vi "AB_820_850_Project_DLL_Info.vi"(7 "action":T1, 8 "error in (no error)":errorcluster, 10 "Dll_info in":T2, 11 "Object In":T3) -> (0 "error out":errorcluster, 2 "Dll info out":T2, 3 "Object Out":T3)   [LabVIEW 2020]
uses:
  <resource>/Framework/Providers/API/ItemRef.ctl
  <vilib>/AppBuilder/RW_Project/AB_RW_Project_PropBag_Action.ctl
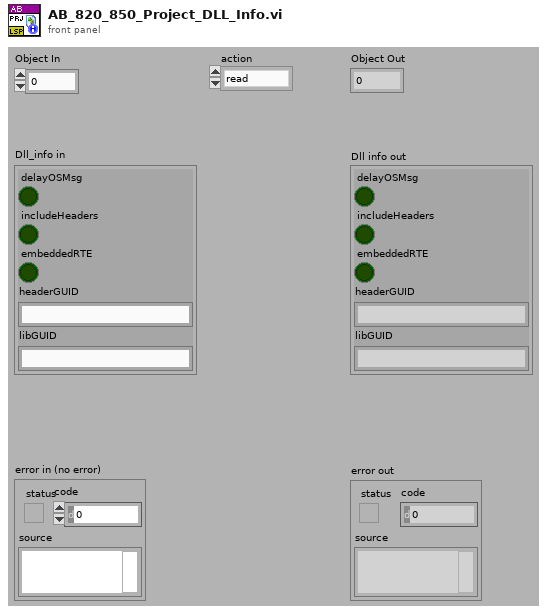
[diagram p1: front panel]
types:
  T1 = typedef "AB_RW_Project_PropBag_Action.ctl" = enum16{"read", "write", "clear", "readPrevious", "writePrevious", "clearPrevious"}
  T2 = cluster{"delayOSMsg":bool, "includeHeaders":bool, "embeddedRTE":bool, "headerGUID":string, "libGUID":string}
  T3 = typedef "ItemRef.ctl" = u64
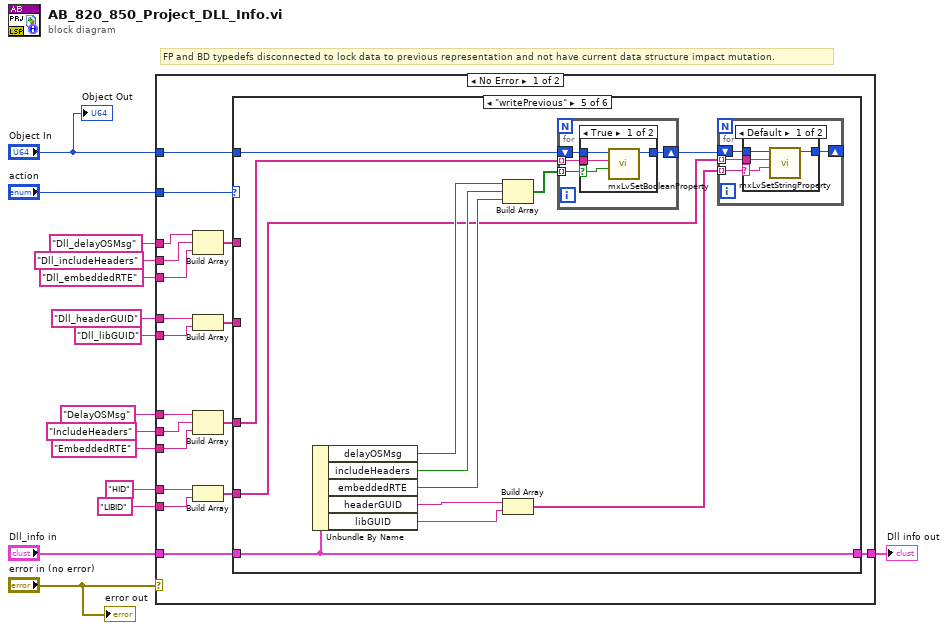
[diagram p0: block diagram]
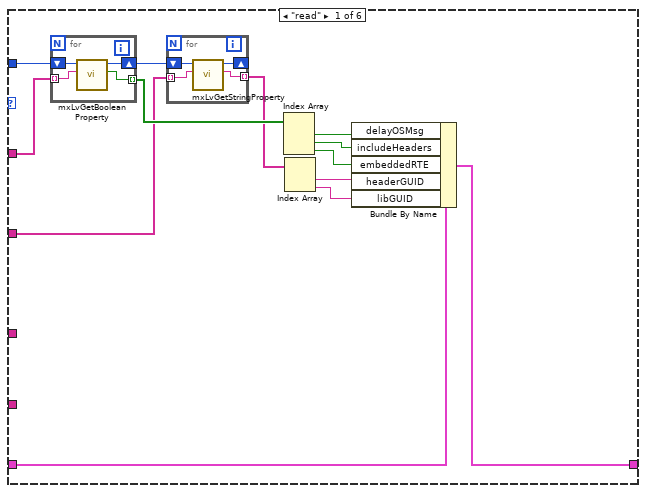
[diagram p2: hidden frame]
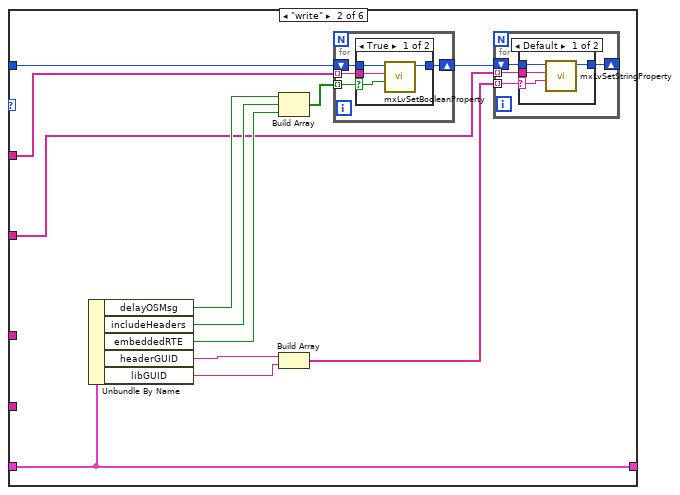
[diagram p3: hidden frame]
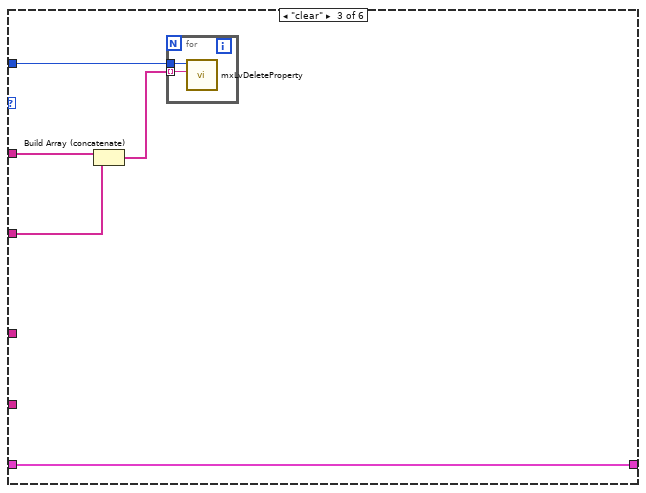
[diagram p6: hidden frame]
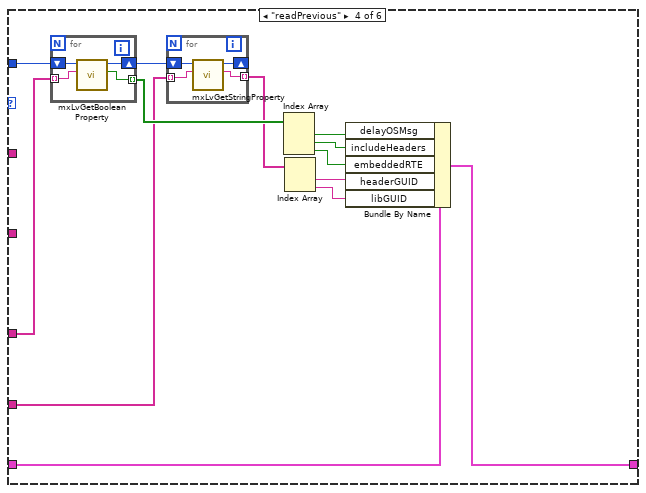
[diagram p7: hidden frame]
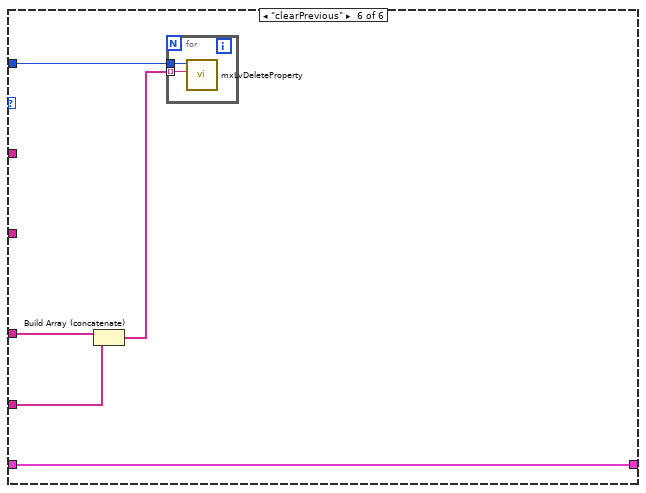
[diagram p10: hidden frame]
diagram:
  # "FP and BD typedefs disconnected to lock data to previous representation and not have current data structure impact mutation."
  n1 = case shown="No Error" "error in (no error)" {
    tunnel: "Object In" -> [w32 _]
    tunnel: [w33 _] -> w13
    tunnel: "Dll_info in" -> [w31 _]
    tunnel: "action" -> [w30 _]
    tunnel: "DelayOSMsg" -> [w29 _]
    tunnel: "IncludeHeaders" ("Tag") -> [w28 _]
    tunnel: "EmbeddedRTE" ("Tag") -> [w27 _]
    tunnel: "HID" -> [w25 _]
    tunnel: "LIBID" -> [w24 _]
    tunnel: "Dll_delayOSMsg" -> [w22 _]
    tunnel: "Dll_includeHeaders" ("Tag") -> [w21 _]
    tunnel: "Dll_embeddedRTE" ("Tag") -> [w20 _]
    tunnel: "Dll_headerGUID" -> [w19 _]
    tunnel: "Dll_libGUID" -> [w18 _]
    frame No Error {
      n2 = Build Array(w22, w21, w20) -> (w17:string[])
      n3 = Build Array(w19, w18) -> (w16:string[])
      n4 = Build Array(w29, w28, w27) -> (w26:string[])
      n5 = Build Array(w25, w24) -> (w23:string[])
      n6 = case shown="\"writePrevious\"" w30 {
        tunnel: [w34 w57 w89 w104 w124 w147] -> w33
        tunnel: w32 -> [w38 w58 w88 w100 w123 w146]
        tunnel: w31 -> [w35 w57 w89 w103 w124 w147]
        tunnel: w26 -> [_ _ _ w101 w122 w144]
        tunnel: w23 -> [_ _ _ w95 w114 w143]
        tunnel: w17 -> [w37 w56 w86 _ _ _]
        tunnel: w16 -> [w36 w55 w85 _ _ _]
        frame "read" {
          n7 = for {
            shift-right: [w53] -> w46
            shift-left: w38 -> [w54]
            tunnel: [w52] -> w45 mode=indexing
            tunnel: w37 -> [w51] mode=indexing
            n8 = call <resource>:"mxLvGetBooleanProperty.vi"("Tag"=w51, "Item"=w54) -> ("Value"=w52:bool, "Item"=w53:T3)  [unwired: 7 in, 1 out]
          }
          n9 = for {
            shift-right: [w49] -> _
            shift-left: w46 -> [w50]
            tunnel: [w48] -> w41 mode=indexing
            tunnel: w36 -> [w47] mode=indexing
            n10 = call <resource>:"mxLvGetStringProperty.vi"("Tag"=w47, "Item"=w50) -> ("Value"=w48:string, "Item"=w49:T3)  [unwired: 7 in, 1 out]
          }
          n11 = Index Array(array=w45) -> (element #1=w44:bool, element #2=w43:bool, element #3=w42:bool)  [unwired: 3 in]
          n12 = Index Array(array=w41) -> (element #1=w40:string, element #2=w39:string)  [unwired: 2 in]
          n13 = Bundle By Name(cluster=w35, "delayOSMsg"=w44, "includeHeaders"=w43, "embeddedRTE"=w42, "headerGUID"=w40, "libGUID"=w39) -> (w34:T2)
        }
        frame "write" {
          n14 = Unbundle By Name(w57) -> ("delayOSMsg"=w66:bool, "includeHeaders"=w65:bool, "embeddedRTE"=w64:bool, "headerGUID"=w62:string, "libGUID"=w61:string)
          n15 = Build Array(w66, w65, w64) -> (w63:bool[])
          n16 = Build Array(w62, w61) -> (w59:string[])
          n17 = for {
            tunnel: w63 -> [w78] mode=indexing
            shift-right: [w77] -> w60
            shift-left: w58 -> [w79]
            tunnel: w56 -> [w76] mode=indexing
            n18 = case shown="True" w78 {
              selector: w78 -> [w82 _]
              tunnel: w79 -> [w83 w84]
              tunnel: w76 -> [w80 _]
              tunnel: [w81 w84] -> w77
              frame True {
                n19 = call <resource>:"mxLvSetBooleanProperty.vi"("Value (F)"=w82, "Tag"=w80, "Item"=w83) -> ("Item"=w81:T3)  [unwired: 7 in, 1 out]
              }
              frame False {
              }
            }
          }
          n20 = for {
            tunnel: w59 -> [w69] mode=indexing
            shift-right: [w68] -> _
            shift-left: w60 -> [w70]
            tunnel: w55 -> [w67] mode=indexing
            n21 = case shown="Default" w69 {
              selector: w69 -> [w72 _]
              tunnel: w70 -> [w74 w75]
              tunnel: w67 -> [w71 _]
              tunnel: [w73 w75] -> w68
              frame Default {
                n22 = call <resource>:"mxLvSetStringProperty.vi"("Value (\"\")"=w72, "Tag"=w71, "Item"=w74) -> ("Item"=w73:T3)  [unwired: 7 in, 1 out]
              }
              frame "" {
              }
            }
          }
        }
        frame "clear" {
          n23 = Build Array (concatenate)(w86, w85) -> (w87:string[])
          n24 = for {
            tunnel: w88 -> [w91]
            tunnel: w87 -> [w90] mode=indexing
            n25 = call <resource>:"mxLvDeleteProperty.vi"("Tag"=w90, "Item"=w91) -> ()  [unwired: 8 in, 2 out]
          }
        }
        frame "readPrevious" {
          n26 = for {
            shift-right: [w111] -> w102
            shift-left: w100 -> [w112]
            tunnel: [w110] -> w99 mode=indexing
            tunnel: w101 -> [w109] mode=indexing
            n27 = call <resource>:"mxLvGetBooleanProperty.vi"("Tag"=w109, "Item"=w112) -> ("Value"=w110:bool, "Item"=w111:T3)  [unwired: 7 in, 1 out]
          }
          n28 = for {
            shift-right: [w107] -> _
            shift-left: w102 -> [w108]
            tunnel: [w106] -> w94 mode=indexing
            tunnel: w95 -> [w105] mode=indexing
            n29 = call <resource>:"mxLvGetStringProperty.vi"("Tag"=w105, "Item"=w108) -> ("Value"=w106:string, "Item"=w107:T3)  [unwired: 7 in, 1 out]
          }
          n30 = Index Array(array=w99) -> (element #1=w98:bool, element #2=w97:bool, element #3=w96:bool)  [unwired: 3 in]
          n31 = Index Array(array=w94) -> (element #1=w93:string, element #2=w92:string)  [unwired: 2 in]
          n32 = Bundle By Name(cluster=w103, "delayOSMsg"=w98, "includeHeaders"=w97, "embeddedRTE"=w96, "headerGUID"=w93, "libGUID"=w92) -> (w104:T2)
        }
        frame "writePrevious" {
          n33 = Unbundle By Name(w124) -> ("delayOSMsg"=w121:bool, "includeHeaders"=w120:bool, "embeddedRTE"=w119:bool, "headerGUID"=w117:string, "libGUID"=w116:string)
          n34 = Build Array(w121, w120, w119) -> (w118:bool[])
          n35 = Build Array(w117, w116) -> (w113:string[])
          n36 = for {
            tunnel: w118 -> [w136] mode=indexing
            shift-right: [w135] -> w115
            shift-left: w123 -> [w137]
            tunnel: w122 -> [w134] mode=indexing
            n37 = case shown="True" w136 {
              selector: w136 -> [w140 _]
              tunnel: w137 -> [w141 w142]
              tunnel: w134 -> [w138 _]
              tunnel: [w139 w142] -> w135
              frame True {
                n38 = call <resource>:"mxLvSetBooleanProperty.vi"("Value (F)"=w140, "Tag"=w138, "Item"=w141) -> ("Item"=w139:T3)  [unwired: 7 in, 1 out]
              }
              frame False {
              }
            }
          }
          n39 = for {
            tunnel: w113 -> [w127] mode=indexing
            shift-right: [w126] -> _
            shift-left: w115 -> [w128]
            tunnel: w114 -> [w125] mode=indexing
            n40 = case shown="Default" w127 {
              selector: w127 -> [w130 _]
              tunnel: w128 -> [w132 w133]
              tunnel: w125 -> [w129 _]
              tunnel: [w131 w133] -> w126
              frame Default {
                n41 = call <resource>:"mxLvSetStringProperty.vi"("Value (\"\")"=w130, "Tag"=w129, "Item"=w132) -> ("Item"=w131:T3)  [unwired: 7 in, 1 out]
              }
              frame "" {
              }
            }
          }
        }
        frame "clearPrevious" {
          n42 = Build Array (concatenate)(w144, w143) -> (w145:string[])
          n43 = for {
            tunnel: w146 -> [w149]
            tunnel: w145 -> [w148] mode=indexing
            n44 = call <resource>:"mxLvDeleteProperty.vi"("Tag"=w148, "Item"=w149) -> ()  [unwired: 8 in, 2 out]
          }
        }
      }
    }
    frame Error {
    }
  }
  "Dll info out" <- w13
  "Object Out" <- "Object In"
  "error out" <- "error in (no error)"
